vi "配置文件write.vi"(7 "updateconfiguration":T1={"主机"="27.154.58.30", "用户"="update", "密码"="std23506", "远程路径"="数据传输系统\\平台数据传输系统.exe", "下载文件名"="数据传输系统.exe", "软件版本"=""}, 8 "error in (no error)":errorcluster caption="错误输入（无错误）", 9 "configuration file path":path caption="配置文件的路径", 10 "键数组":string[](array[string]), 11 "段":string="应用程序交互") -> (0 "error out":errorcluster caption="错误输出")   [LabVIEW 2016, in "数据传输系统-05.lvlib" / "自动更新.lvlib"]
uses:
  <vilib>/Utility/config.llb/Write Key (I32).vi
  <vilib>/Utility/config.llb/Write Key (String).vi
  <vilib>/Utility/config.llb/NI_LVConfig.lvlib
  <vilib>/Utility/Data Type/NI_Data Type.lvlib
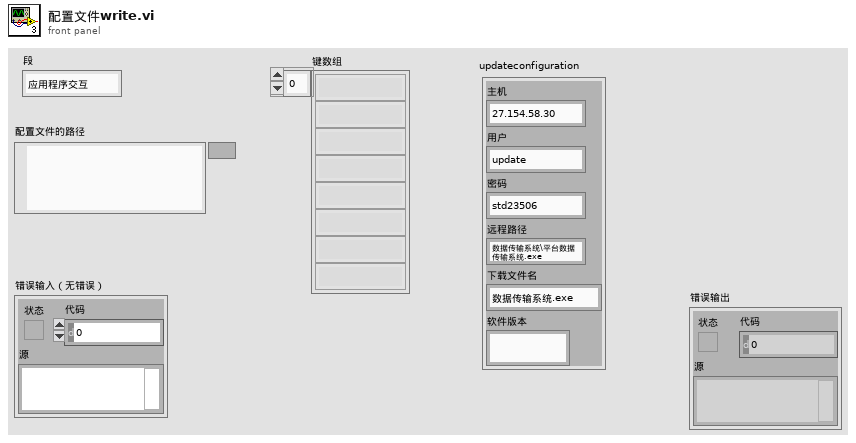
[diagram p1: front panel]
types:
  T1 = cluster{"主机":string, "用户":string, "密码":string, "远程路径":string, "下载文件名":string, "软件版本":string}
  T2 = typedef "NI_LVConfig.lvlib/Config Data RefNum.ctl" = refnum<k1>
  T3 = typedef "NI_Data Type.lvlib/Data Type.ctl" = enum8{"Invalid Type", "Void", "I8", "I16", "I32", "I64", "U8", "U16", "U32", "U64", "Single Float", "Double Float", "Extended Float", "Single Complex", "Double Complex", "Extended Complex", "Enum U8", "Enum U16", "Enum U32", "Enum U64", "Single Float With Unit", "Double Float With Unit", "Extended Float With Unit", "Single Complex with Unit", "Double Complex with Unit", "Extended Complex with Unit", "Boolean", "String", "Path", "Picture", "Tag", "Array", "Cluster", "Variant", "LV Variant", "Waveform", "Timestamp", "Digital Waveform", "Digital Data", "ExpressData", "Refnum", "External Data", "VI", "Poly VI", "LabVIEW Class Instance", "Fixed Point"}
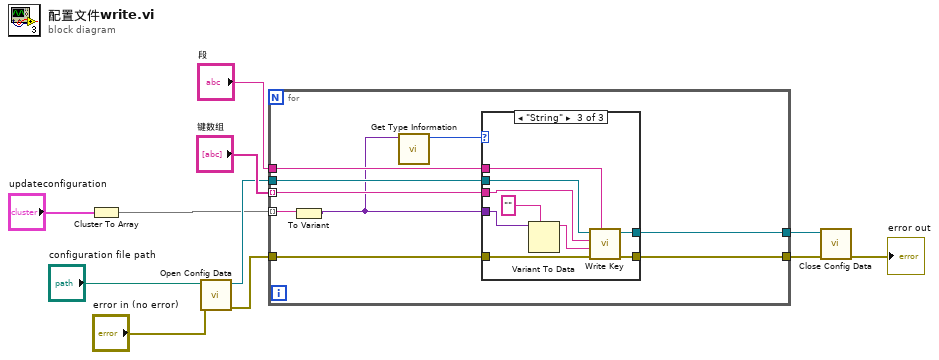
[diagram p0: block diagram]
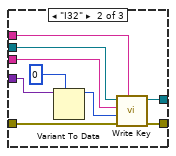
[diagram p3: hidden frame]
diagram:
  n1 = Cluster To Array(cluster="updateconfiguration") -> (array=w2:string[])
  n2 = call <vilib>:"Open Config Data.vi"("error in (no error)"="error in (no error)", "configuration file path"="configuration file path") -> ("error out"=w8:errorcluster, "refnum"=w9:T2)  [unwired: 7 in, 1 out]
  n3 = for {
    tunnel: "键数组" -> [w16] mode=indexing
    tunnel: w2 -> [w13] mode=indexing
    tunnel: w9 -> [w19]
    tunnel: w8 -> [w18]
    tunnel: "段" -> [w17]
    tunnel: [w15] -> w6
    tunnel: [w14] -> w5
    n4 = To Variant(anything=w13) -> (Variant=w12:variant)
    n5 = call <vilib>:"Get Type Information.vi"("Variant"=w12) -> ("Type"=w20:T3)  [unwired: 6 in, 4 out]
    n6 = case shown="\"String\"" w20 {
      tunnel: [w22 w29 w38] -> w15
      tunnel: [w21 w28 w37] -> w14
      tunnel: w12 -> [_ w23 w36]
      tunnel: w19 -> [w22 w27 w35]
      tunnel: w18 -> [w21 w26 w34]
      tunnel: w17 -> [_ w25 w33]
      tunnel: w16 -> [_ w24 w32]
      frame "Invalid Type", Default {
      }
      frame "I32" {
        n7 = Variant To Data(type=0, Variant=w23) -> (data=w30:i32)  [unwired: 1 in, 1 out]
        n8 = call-poly <vilib>:"Write Key.vi"("section"=w25, "error in (no error)"=w26, "value"=w30, "key"=w24, "refnum"=w27) -> ("error out"=w28:errorcluster, "refnum out"=w29:T2)  [unwired: 4 in, 1 out]
      }
      frame "String" {
        n9 = Variant To Data(type="", Variant=w36) -> (data=w39:string)  [unwired: 1 in, 1 out]
        n10 = call-poly <vilib>:"Write Key.vi"("section"=w33, "error in (no error)"=w34, "value"=w39, "key"=w32, "refnum"=w35) -> ("error out"=w37:errorcluster, "refnum out"=w38:T2)  [unwired: 4 in, 1 out]
      }
    }
  }
  n11 = call <vilib>:"Close Config Data.vi"("error in (no error)"=w5, "refnum"=w6) -> ("error out"=→"error out":errorcluster)  [unwired: 8 in, 1 out]
